vi "Error43.vi"(8 "error in":errorcluster={"status"=TRUE, "code"=43, "source"=""}) -> (0 "error out":errorcluster)   [LabVIEW 2014]
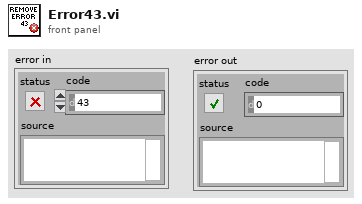
[diagram p1: front panel]
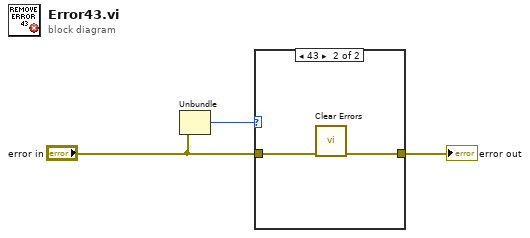
[diagram p0: block diagram]
diagram:
  n1 = Unbundle("error in") -> ("code"=w3:i32)  [unwired: 2 out]
  n2 = case shown="43" w3 {
    tunnel: "error in" -> [w4 w6]
    tunnel: [w4 w5] -> w2
    frame Default {
    }
    frame 43 {
      n3 = call <vilib>:"Clear Errors.vi"("error in (no error)"=w6) -> ("error out"=w5:errorcluster)  [unwired: 5 in, 1 out]
    }
  }
  "error out" <- w2
